vi "Gyro PID Back C2 Stop.vi"(6 "Target angle":sgl, 7 "Threshold to Color":i32=1200, 8 "Threshold to slow":i32=1000, 9 "Min. speed":i32=20, 10 "Max. speed":i32=40, 11 "EV3 in":T1) -> (3 "EV3 out":T1)   [LabVIEW 2016]
uses:
  <vilib>/NXT/Subs/LVHSConnector.ctl
  <vilib>/NXT/LegoClasses/BrickReference/BrickReference.lvclass
  <vilib>/NXT/Block Support/NXT_OutputPort.ctl
  <vilib>/NXT/Block Support/NXT_InputPort.ctl
  <vilib>/NXT/NXTIO Xnodes/NXTIONodeSubVIs/LEGOResetMotors.vi
  <vilib>/NXT/Dual Mode Library/Motors/Rotation.vi
  <vilib>/NXT/Dual Mode Library/Sensors/EV3_Color_Reflect.vi
  <vilib>/NXT/NXTIO Xnodes/NXTIONodeSubVIs/NXTMotorSteeringOn.vi
  <vilib>/NXT/NXTIO Xnodes/NXTIONodeSubVIs/NXTStopMotors.vi
  <vilib>/NXT/Dual Mode Library/Waits/Wait_Num.vi
  <vilib>/NXT/NXTIO Xnodes/NXTIOXNode/NXTIO.xnode
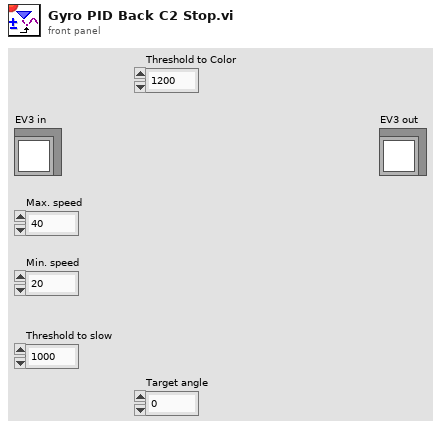
[diagram p1: front panel]
types:
  T1 = typedef "LVHSConnector.ctl" = refnum<class "BrickReference.lvclass">
  T2 = typedef "NXT_OutputPort.ctl" = u8
  T3 = typedef "NXT_InputPort.ctl" = u32
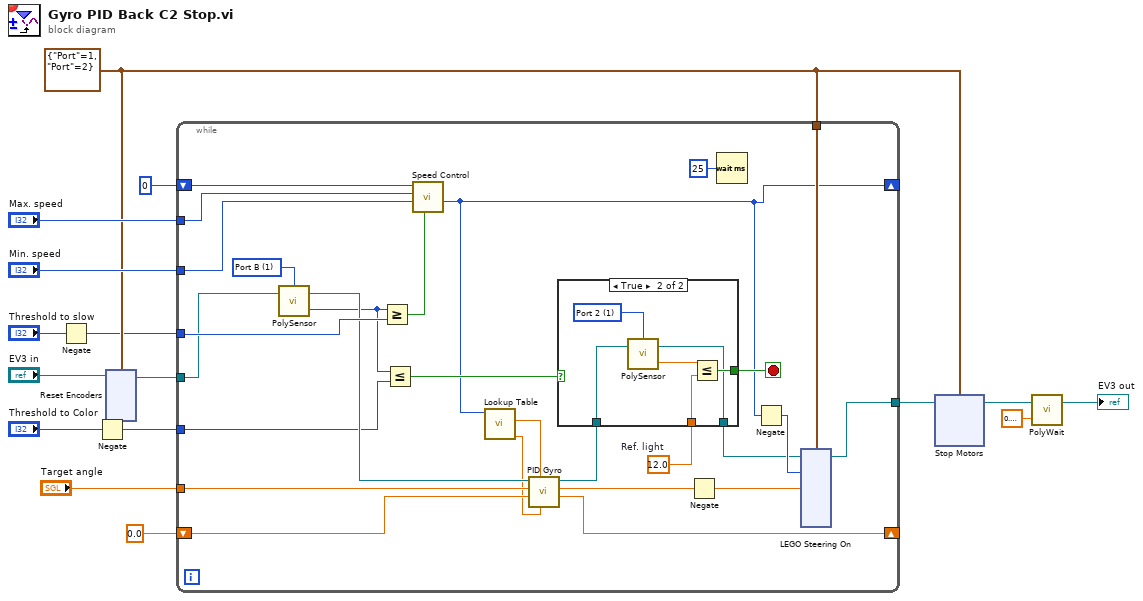
[diagram p0: block diagram]
diagram:
  w6 = cluster{"Port":T2, "Port":T2} {"Port"=1, "Port"=2} ("Motor")
  n1 = Negate(x="Threshold to slow") -> (-x=w2:i32)
  n2 = Negate(x="Threshold to Color") -> (-x=w1:i32)
  n3 = xnode "Reset Encoders"("Motors"=w6, "NXT/EV3"="EV3 in") -> ("NXT/EV3"=w12:T1)
  n4 = while {
    tunnel: w12 -> [w32]
    shift-right: [w43] -> _
    shift-left: sgl 0.0 -> [w28]
    tunnel: "Target angle" -> [w42]
    tunnel: [w39] -> w8
    tunnel: w6 -> [w41]
    shift-right: [w19] -> _
    shift-left: 0 -> [w36]
    tunnel: "Min. speed" -> [w33]
    tunnel: "Max. speed" -> [w35]
    tunnel: w2 -> [w34]
    tunnel: w1 -> [w27]
    stop <- w20 stop-if-true
    w21 = sgl 12.0  # Ref. light
    w40 = T2 1 items=["Port A", "Port B", "Port C", "Port D"] ("Port (Port A)")
    n5 = call-poly <vilib>:"PolySensor.vi"("NXT/EV3"=w32, "Port (Port A)"=w40) -> ("Angle of Rotation"=w29:i32, "NXT/EV3"=w31:T1)  [unwired: 1 in]
    n6 = Greater Or Equal?(x=w29, y=w34) -> (x >= y?=w30:bool)
    n7 = Less Or Equal?(x=w29, y=w27) -> (x <= y?=w24:bool)
    n8 = call "Speed Control.vi"("Speed Up or Down?"=w30, "Min. speed"=w33, "Max. speed"=w35, "Ini. speed"=w36) -> ("Speed out"=w19:i32)  [unwired: 7 in]
    n9 = call "Lookup Table.vi"("Speed"=w19) -> ("I"=w17:dbl, "P"=w18:dbl)  [unwired: 9 in]
    n10 = call "PID Gyro.vi"("K_i"=w17, "K_p"=w18, "Previous integral"=w28, "Target angle"=w42, "EV3 in"=w31) -> ("New integral"=w43:sgl, "Total error"=w37:sgl, "EV3 out"=w23:T1)  [unwired: 4 in]
    n11 = case shown="True" w24 {
      tunnel: [_ w48] -> w20
      tunnel: w23 -> [w44 w47]
      tunnel: [w44 w46] -> w22
      tunnel: w21 -> [_ w45]
      frame False {
      }
      frame True {
        w50 = T3 1 items=["Port 1", "Port 2", "Port 3", "Port 4"] ("Port (Port 1)")
        n12 = call-poly <vilib>:"PolySensor.vi"("NXT/EV3"=w47, "Port (Port 1)"=w50) -> ("Scaled Value"=w49:sgl, "NXT/EV3"=w46:T1)  [unwired: 1 in]
        n13 = Less Or Equal?(x=w49, y=w45) -> (x <= y?=w48:bool)
      }
    }
    n14 = Negate(x=w37) -> (-x=w25:sgl)
    n15 = Wait (ms)(milliseconds to wait=u32 25) -> ()  [unwired: 1 out]
    n16 = Negate(x=w19) -> (-x=w26:i32)
    n17 = xnode "LEGO Steering On"("Steering 1"=w25, "Power 1"=w26, "Motors"=w41, "NXT/EV3"=w22) -> ("NXT/EV3"=w39:T1)
  }
  n18 = xnode "Stop Motors"("Motors"=w6, "NXT/EV3"=w8) -> ("NXT/EV3"=w7:T1)
  n19 = call-poly <vilib>:"PolyWait.vi"("Time (1 sec)"=sgl 0.2, "NXT/EV3"=w7) -> ("NXT/EV3"=→"EV3 out":T1)  [unwired: 2 in]
